vi "normalize_vector_array_single.vi"(1 "2 element vector":sgl[](array[numeric])) -> (0 "normalized vector out":sgl[](array[numeric]))   [LabVIEW 2019]
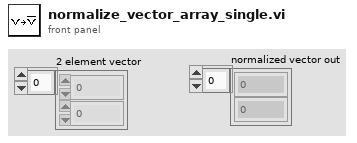
[diagram p1: front panel]
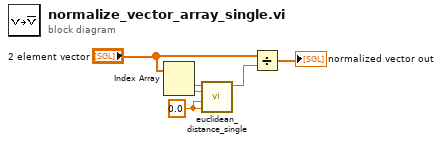
[diagram p0: block diagram]
diagram:
  w6 = sgl 0.0
  n1 = Index Array(array="2 element vector") -> (element #1=w4:sgl, element #2=w3:sgl)  [unwired: 2 in]
  n2 = call "euclidean_distance_single.vi"("Point 2 Y"=w6, "Point 2 X"=w6, "Point 1 Y"=w3, "Point 1 X"=w4) -> ("Distance"=w5:sgl)  [unwired: 7 in]
  n3 = Divide(x="2 element vector", y=w5) -> (x/y=→"normalized vector out":sgl[])
